vi "FRCts20_WebMethods_Comment_GET.vi"(7 "httpRequestID":u32, 10 "comment":string, 11 "request":string) -> ()   [LabVIEW 2014, in "FRCts20_WebMethods.lvlib"]
doc: "<B>GET</B> on the specified <B>comment</B> resource\n\nIf comment is not specified, will return all resources.\n\nhttp://<server address>:<port>/FRCts/request/<B>request</B>/comment/<B>comment</B>"
uses:
  FRCts20_WebMethods.lvlib
  <vilib>/wsapi/NI_WebServices.lvlib
  Backend/source/VI Source/FRCts20_Backend_API/FRCts20_Backend_API_Comment.vi
  Backend/source/VI Source/FRCts20_Backend_API/FRCts20_Backend_API_Note.ctl
  Backend/source/VI Source/FRCts20_Backend_API/FRCts20_Backend_API_Status.ctl
  Backend/source/VI Source/FRCts20_Backend_API/FRCts20_Backend_API_Request.ctl
  Backend/source/VI Source/FRCts20_Backend_API/FRCts20_Backend_API_Request.vi
  Backend/source/VI Source/FRCts20_Backend_API/FRCts20_Backend_API_Command_Request.ctl
  Backend/source/VI Source/FRCts20_Backend_API/FRCts20_Backend_API_Command_Note.ctl
  Controls/FRCts20_WebMethods_ctl_returntype.ctl
panel:
  in  "query":string
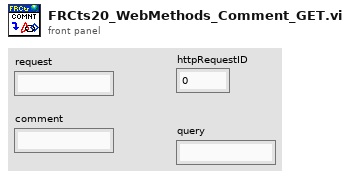
[diagram p1: front panel]
types:
  T1 = typedef "FRCts20_Backend_API.lvlib/FRCts20_Backend_API_Command_Note.ctl" = string
  T2 = typedef "FRCts20_Backend_API.lvlib/FRCts20_Backend_API_Note.ctl" = cluster{"Note Index":u32, "Request Index":u32, "Author":string, "Time Entered":timestamp, "Text":string, "Solution":bool, "APIReturn":string}
  T3 = typedef "FRCts20_Backend_API.lvlib/FRCts20_Backend_API_Command_Request.ctl" = string
  T4 = typedef "FRCts20_Backend_API.lvlib/FRCts20_Backend_API_Request.ctl" = cluster{"Request Index":u32, "Description":string, "Status":T5, "Open Date":timestamp, "Last Update":timestamp, "Closed Date":timestamp, "Notes":cluster{"Note Index":u32, "Text":string, "Time Entered":timestamp, "Author":string, "Solution":bool}[], "Team Index":u32, "APIReturn":string}
  T5 = typedef "FRCts20_Backend_API.lvlib/FRCts20_Backend_API_Status.ctl" = enum16{"Open", "In Work", "Closed"}
  T6 = typedef "FRCts20_WebMethods.lvlib/FRCts20_WebMethods_ctl_returntype.ctl" = string
  T7 = cluster{"Notes":cluster{"Note Index":u32, "Text":string, "Soln?":bool}[]}
  T8 = cluster{"Note Index":u32, "Text":string, "Time Entered":timestamp, "Author":string, "Solution":bool}[]
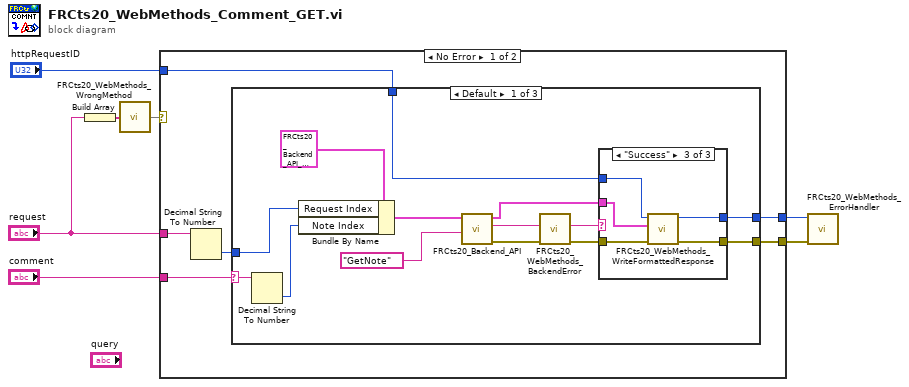
[diagram p0: block diagram]
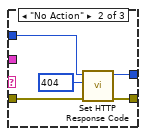
[diagram p3: hidden frame]
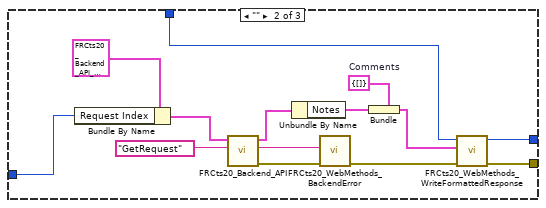
[diagram p4: hidden frame]
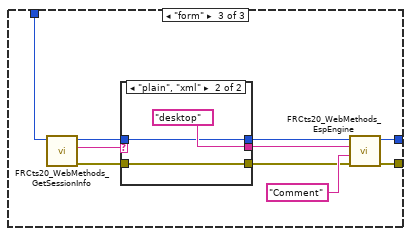
[diagram p5: hidden frame]
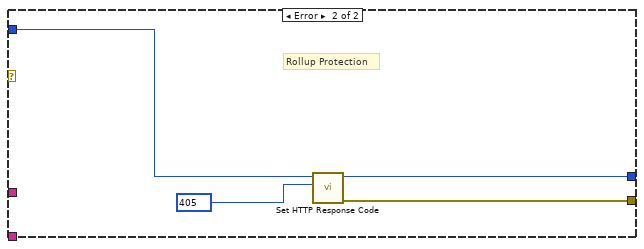
[diagram p7: hidden frame]
diagram:
  n1 = Build Array("request") -> (w6:string[])
  n2 = call "FRCts20_WebMethods_WrongMethod.vi"(4:w6) -> (1:w7)  [unwired: 3 in, 1 out]
  n3 = case shown="No Error" w7 {
    tunnel: "httpRequestID" -> [w11 w73]
    tunnel: [w12 w71] -> w3
    tunnel: [w13 w70] -> w4
    tunnel: "comment" -> [w8 _]
    tunnel: "request" -> [w10 _]
    frame No Error {
      n4 = Decimal String To Number(string=w10) -> (number=w9:i32)  [unwired: 2 in, 1 out]
      n5 = case shown="Default" w8 {
        selector: w8 -> [w14 _ _]
        tunnel: [w27 w53 w56] -> w13
        tunnel: [w26 w52 w55] -> w12
        tunnel: w11 -> [w21 w47 w54]
        tunnel: w9 -> [w16 w45 _]
        frame Default {
          n6 = Decimal String To Number(string=w14) -> (number=w17:i32)  [unwired: 2 in, 1 out]
          n7 = Bundle By Name(cluster=T2 {"Note Index"=0, "Request Index"=0, "Author"="", "Time Entered"=timestamp(0 s since 1904-01-01), "Text"="", "Solution"=FALSE, "APIReturn"=""} ("Note In"), "Request Index"=w16, "Note Index"=w17) -> (w18:T2)
          n8 = call-poly "FRCts20_Backend_API.vi"("Command"=T1 "GetNote", "Note In"=w18) -> ("error out"=w25:errorcluster, "Status"=w20:string, "Note Out"=w22:T2)  [unwired: 7 in]
          n9 = call "FRCts20_WebMethods_BackendError.vi"("error in (no error)"=w25, "Status"=w20) -> ("error out"=w24:errorcluster, "Status out"=w23:string)  [unwired: 8 in]
          n10 = case shown="\"Success\"" w23 {
            tunnel: [w28 w34 w39] -> w27
            tunnel: [w29 w33 w38] -> w26
            tunnel: w24 -> [w28 w32 w37]
            tunnel: w22 -> [_ _ w36]
            tunnel: w21 -> [w29 w31 w35]
            frame "Backend Error", Default {
            }
            frame "No Action" {
              w30 = 404 items=["100"=100, "101"=101, "200"=200, "201"=201, "202"=202, "203"=203, "204"=204, "205"=205, "206"=206, "300"=300, "301"=301, "302"=302, "303"=303, "304"=304, "305"=305, "306"=306, "307"=307, "400"=400, "401"=401, "402"=402, "403"=403, "404"=404, "405"=405, "406"=406, "407"=407, "408"=408, "409"=409, "410"=410, "411"=411, "412"=412, "413"=413, "414"=414, "415"=415, "416"=416, "417"=417, "500"=500, "501"=501, "502"=502, "503"=503, "504"=504, "505"=505] ("response code (200)")
              n11 = call <vilib>:"Set HTTP Response Code.vi"("error in (no error)"=w32, "response code (200)"=w30, "httpRequestID"=w31) -> ("error out"=w34:errorcluster, "httpRequestID out"=w33:u32)  [unwired: 7 in]
            }
            frame "Success" {
              n12 = call "FRCts20_WebMethods_WriteFormattedResponse.vi"("error in (no error)"=w37, "Response Cluster"=w36, "httpRequestID"=w35) -> ("error out"=w39:errorcluster, "httpRequestID out"=w38:u32)  [unwired: 7 in]
            }
          }
        }
        frame "" {
          w40 = T7 {"Notes"=[]}  # Comments
          n13 = Bundle By Name(cluster=T4 {"Request Index"=0, "Description"="", "Status"=enum."Open", "Open Date"=timestamp(0 s since 1904-01-01), "Last Update"=timestamp(0 s since 1904-01-01), "Closed Date"=timestamp(0 s since 1904-01-01), "Notes"=[], "Team Index"=0, "APIReturn"=""} ("Request"), "Request Index"=w45) -> (w44:T4)
          n14 = call-poly "FRCts20_Backend_API.vi"("Command"=T3 "GetRequest", "Request In"=w44) -> ("error out"=w50:errorcluster, "Status"=w49:string, "Request Out"=w48:T4)  [unwired: 7 in]
          n15 = Unbundle By Name(w48) -> ("Notes"=w42:T8)
          n16 = call "FRCts20_WebMethods_BackendError.vi"("error in (no error)"=w50, "Status"=w49) -> ("error out"=w51:errorcluster)  [unwired: 8 in, 1 out]
          n17 = Bundle(cluster=w40, "Notes"=w42) -> (w41:T7)
          n18 = call "FRCts20_WebMethods_WriteFormattedResponse.vi"("error in (no error)"=w51, "Response Cluster"=w41, "httpRequestID"=w47) -> ("error out"=w53:errorcluster, "httpRequestID out"=w52:u32)  [unwired: 7 in]
        }
        frame "form" {
          n19 = call "FRCts20_WebMethods_GetSessionInfo.vi"("httpRequestID"=w54) -> ("error out"=w61:errorcluster, "Return Type"=w62:T6, "httpRequestID out"=w60:u32)  [unwired: 8 in]
          n20 = case shown="\"plain\", \"xml\"" w62 {
            selector: w62 -> [w65 _]
            tunnel: w61 -> [w66 w68]
            tunnel: w60 -> [w64 w67]
            tunnel: [w66 w68] -> w59
            tunnel: [w65 T6 "desktop" ("Return Type")] -> w58
            tunnel: [w64 w67] -> w57
            frame Default {
            }
            frame "plain", "xml" {
            }
          }
          n21 = call "FRCts20_WebMethods_EspEngine.vi"("error in (no error)"=w59, "Cluster"="Comment", "Return Type"=w58, "httpRequestID"=w57) -> ("error out"=w56:errorcluster, "httpRequestID out"=w55:u32)  [unwired: 6 in]
        }
      }
    }
    frame Error {
      w72 = 405 items=["100"=100, "101"=101, "200"=200, "201"=201, "202"=202, "203"=203, "204"=204, "205"=205, "206"=206, "300"=300, "301"=301, "302"=302, "303"=303, "304"=304, "305"=305, "306"=306, "307"=307, "400"=400, "401"=401, "402"=402, "403"=403, "404"=404, "405"=405, "406"=406, "407"=407, "408"=408, "409"=409, "410"=410, "411"=411, "412"=412, "413"=413, "414"=414, "415"=415, "416"=416, "417"=417, "500"=500, "501"=501, "502"=502, "503"=503, "504"=504, "505"=505] ("response code (200)")
      # "Rollup Protection"
      n22 = call <vilib>:"Set HTTP Response Code.vi"("response code (200)"=w72, "httpRequestID"=w73) -> ("error out"=w70:errorcluster, "httpRequestID out"=w71:u32)  [unwired: 8 in]
    }
  }
  n23 = call "FRCts20_WebMethods_ErrorHandler.vi"("error in"=w4, "LabVIEW Web Service Request"=w3) -> ()  [unwired: 8 in, 2 out]
